vi "Write.vi"(0 "element":cluster{timestamp[], dbl[]}[](array[cluster])) -> (1 "previous element":cluster{timestamp[], dbl[]}[](array[cluster]), 2 "channel":T1)   [LabVIEW 2020, in "Tag-a[.](c(a[.](stamp),a[.](dbl))).lvlib"]
doc: "Writes a value to a Tag channel."
uses:
  <extravilib>/ChannelInstances/Tag-a[.](c(a[.](stamp),a[.](dbl))).lvlib
  <extravilib>/ChannelInstances/Tag-a[.](c(a[.](stamp),a[.](dbl)))/))Channel.ctl
  <extravilib>/ChannelInstances/Tag-a[.](c(a[.](stamp),a[.](dbl)))/Endpoint.vi
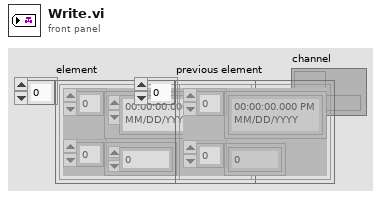
[diagram p1: front panel]
types:
  T1 = typedef "Tag-a[.](c(a[.](stamp),a[.](dbl))).lvlib/))Channel.ctl" = refnum<queue>
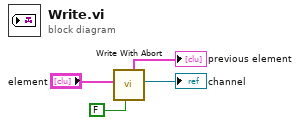
[diagram p0: block diagram]
diagram:
  n1 = call <extravilib>:"Write With Abort.vi"("abort"=FALSE, "element"="element") -> ("channel"=→"channel":T1, "previous element"=→"previous element":cluster{timestamp[], dbl[]}[])  [unwired: 7 in, 1 out]
